vi "interface in.vi"(7 "manual control":refnum<vi>) -> (4 "time (global)":dbl, 8 "MPV":i32, 10 "manual control":T2, 15 "global stop":bool)   [LabVIEW 2010]
uses:
  Licor-Sequences.ctl
  Johnny/pertrasgc fpga/GVUTC.vi
  Johnny/pertrasgc fpga/gvbooleschRT.vi
  Johnny/pertrasgc fpga/GVZeitenZyklen.vi
  Johnny/pertrasgc fpga/GVVentilposition.vi
panel:
  out "Numerisch":i32
  in  "manual control":T2={"sequence manual"=enum."WAIT", "sequence manual ?"=FALSE}
  out "sequence manual":T1=enum."WAIT"
  in  "sequence manual":T1=enum."warmup"
  out "sequence manual ?":bool
  in  "sequence manual ?":bool
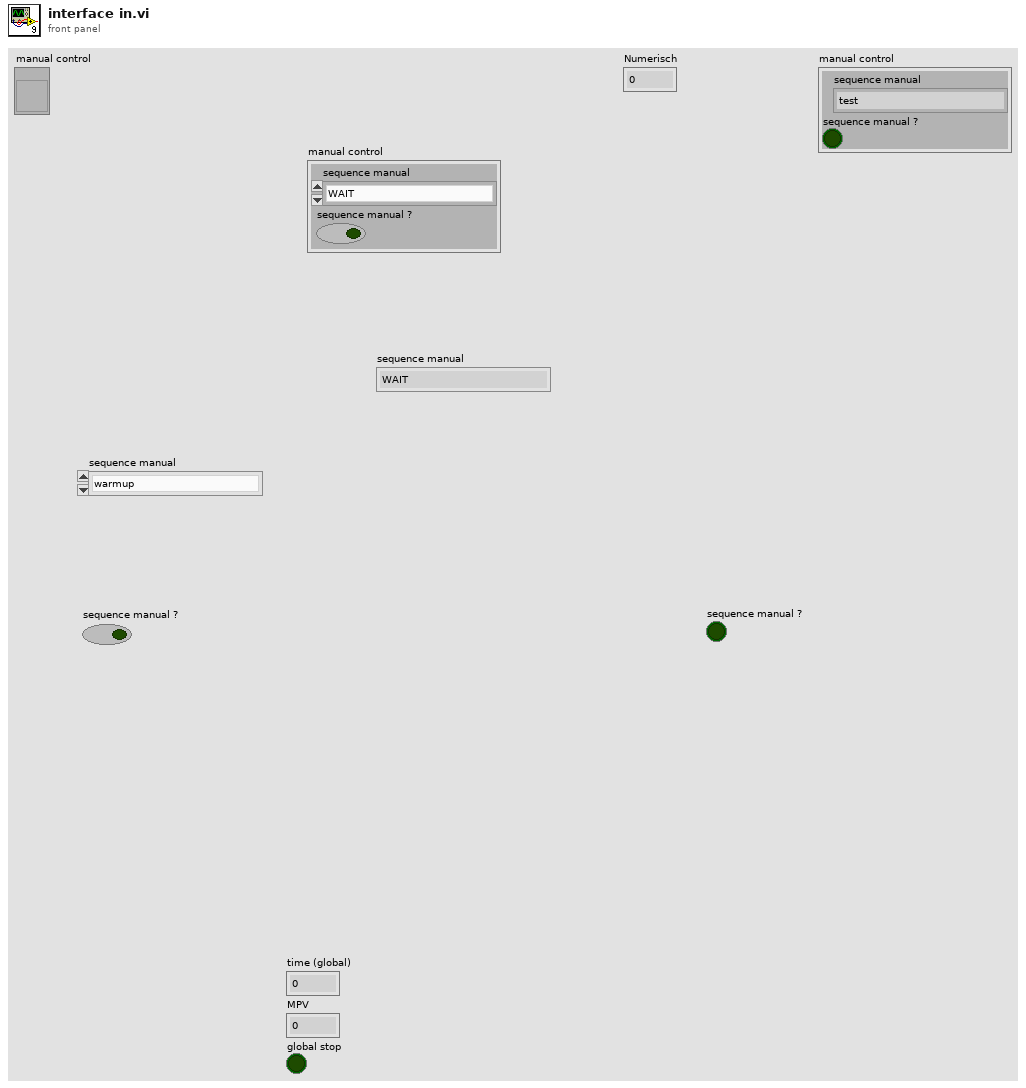
[diagram p1: front panel]
types:
  T1 = typedef "Licor-Sequences.ctl" = enum16{"test", "WAIT", "warmup", "initialize", "calibrate Z", "calibrate S"}
  T2 = cluster{"sequence manual":T1, "sequence manual ?":bool}
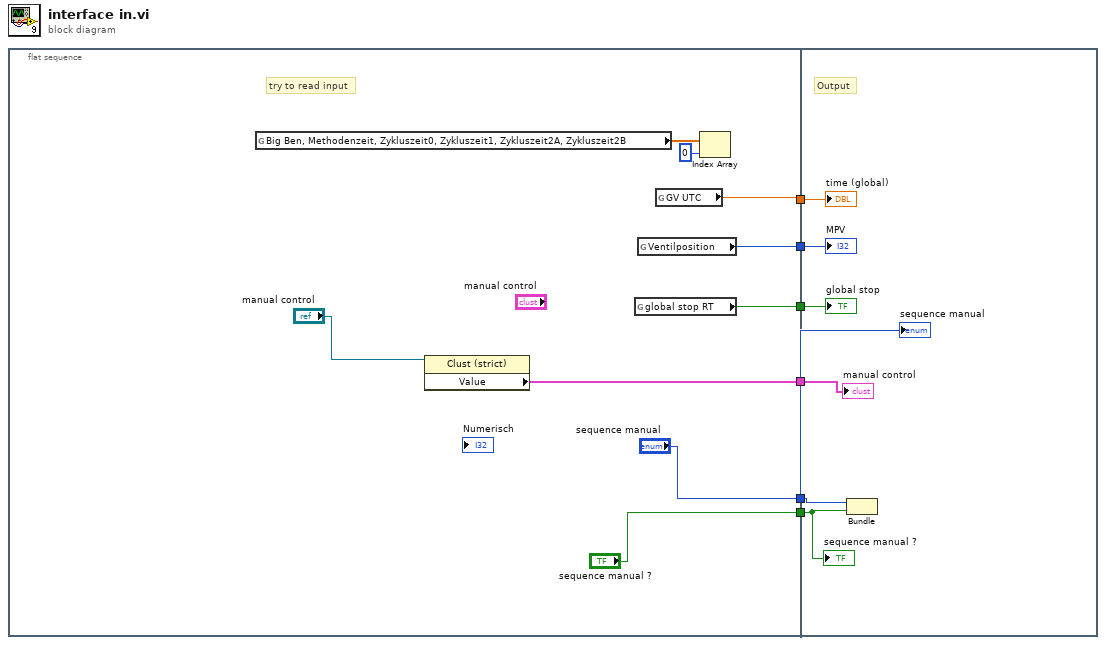
[diagram p0: block diagram]
diagram:
  n1 = flat-sequence {
    tunnel: [w7] -> w6
    tunnel: [w15] -> w5
    tunnel: [w14] -> w4
    tunnel: ["sequence manual"] -> w3
    tunnel: ["sequence manual ?"] -> w2
    tunnel: [w8] -> w1
    tunnel: w6 -> [w20]
    tunnel: w5 -> [w21]
    tunnel: w4 -> [w19]
    tunnel: w3 -> [w18]
    tunnel: w2 -> [w17]
    tunnel: w1 -> [w16]
    frame #0 {
      # "try to read input"
      n2 = global read "GVZeitenZyklen.vi" "Big Ben, Methodenzeit, Zykluszeit0, Zykluszeit1, Zykluszeit2A, Zykluszeit2B"() -> (w12:dbl[])
      n3 = property on="Eigenschaftsknoten" class="Clust (strict)"(reference="manual control") -> ("Value"=w8:T2)  [unwired: 1 in, 2 out]
      n4 = global read "gvbooleschRT.vi" "global stop RT"() -> (w14:bool)
      n5 = global read "GVVentilposition.vi" "Ventilposition"() -> (w15:i32)
      n6 = global read "GVUTC.vi" "GV UTC"() -> (w7:dbl)
      n7 = Index Array(array=w12, index=0 ("Index")) -> ()  [unwired: 1 out]
    }
    frame #1 {
      # "Output"
      n8 = Bundle("sequence manual"=w18, "sequence manual ?"=w17) -> ()  [unwired: 1 in, 1 out]
      "time (global)" <- w20
      "MPV" <- w21
      "global stop" <- w19
      "sequence manual ?" <- w17
      "sequence manual" <- w18
      "manual control" <- w16
    }
  }
